vi "Configure Voltage Protection Value.vi"(8 "error in (no error)":errorcluster, 9 "Voltage Protection Value (0)":dbl min=0.0 step=0.1 format="%^#_6g", 10 "Protection Mode (0: Regulation)":u16(ring) items=["Regulation", "Switching"], 11 "VISA resource name":refnum<visa-resource-name>) -> (0 "error out":errorcluster, 3 "VISA resource name out":refnum<visa-resource-name>)   [LabVIEW 2017, in "HH PLI Series.lvlib"]
doc: "Sets a lower voltage protection value."
uses:
  HH PLI Series.lvlib
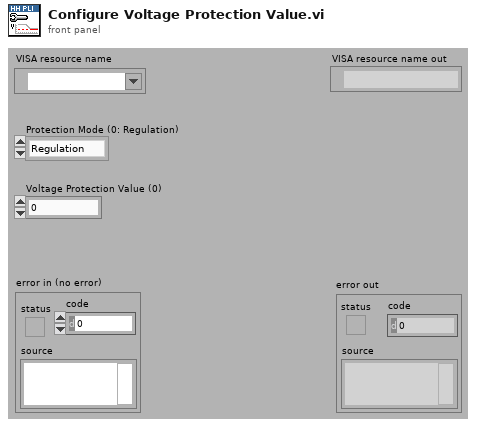
[diagram p1: front panel]
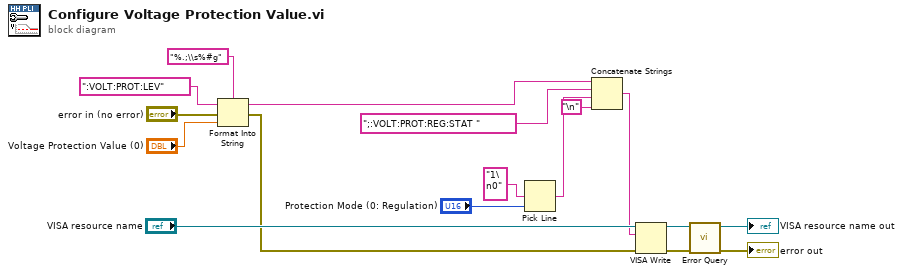
[diagram p0: block diagram]
diagram:
  n1 = Format Into String(format string="%.;\\s%#g", initial string=":VOLT:PROT:LEV", error in="error in (no error)", "Voltage Protection Value (0)") -> (resulting string=w2:string, error out=w1:errorcluster)
  n2 = Pick Line(multi-line string="1\n0", line index="Protection Mode (0: Regulation)") -> (output string=w4:string)  [unwired: 1 in]
  n3 = Concatenate Strings(w2, ";:VOLT:PROT:REG:STAT ", w4, "\n") -> (w8:string)
  n4 = VISA Write(VISA resource name="VISA resource name", write buffer=w8, error in (no error)=w1) -> (VISA resource name out=w12:refnum<visa-resource-name>, error out=w13:errorcluster)  [unwired: 1 out]
  n5 = call "Error Query.vi"("error in (no error)"=w13, "VISA resource name"=w12) -> ("error out"=→"error out":errorcluster, "VISA resource name out"=→"VISA resource name out":refnum<visa-resource-name>)  [unwired: 6 in, 2 out]
